vi "Equivalent Circuit.vi"(0 "VISA resource name":refnum<visa-resource-name>, 1 "Equivalent Circuit (0:A)":u32(ring) items=["A", "B", "C", "D", "E"], 2 "Equivalent Circuit Page (T:Not Displaying)":bool=TRUE, 5 "R (1.0 ohm)":dbl=1.0 min=-1e-36 max=9.99999e+37 format="%^.3e", 7 "L (1,0E-6 H)":dbl=1e-06 min=-1e-36 max=1e+38 format="%^.3e", 9 "Ca (1,0E-6 F)":dbl=1e-06 min=-1e-36 max=1e+38 format="%^.3e", 11 "error in (no error)":errorcluster, 12 "Cb (1,0E-6 F)":dbl=1e-06 max=1e+38 format="%^.3e") -> (4 "VISA resource name out":refnum<visa-resource-name>, 15 "error out":errorcluster)   [LabVIEW 2017, in "Agilent 4194.lvlib"]
doc: "This function sets the equivalent circuit and parameters for this equivalent circuit."
uses:
  Agilent 4194.lvlib
panel:
  # "Not Displaying"
  # "Displaying"
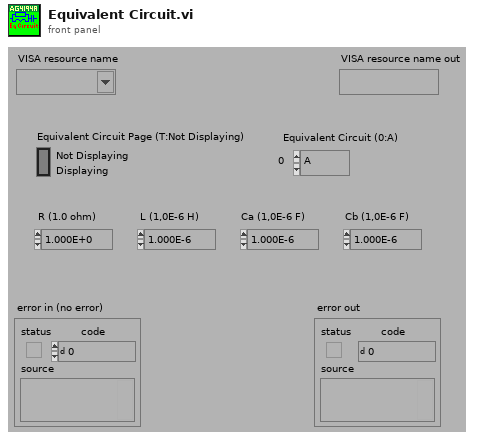
[diagram p1: front panel]
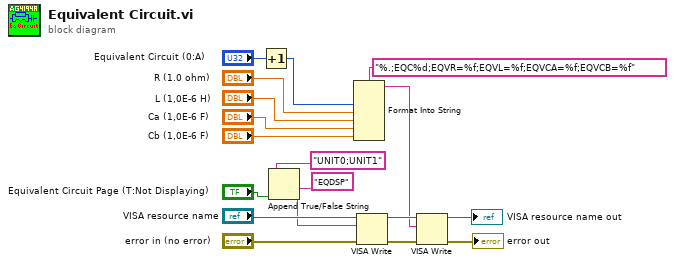
[diagram p0: block diagram]
diagram:
  n1 = Increment(x="Equivalent Circuit (0:A)") -> (x+1=w3:u32)
  n2 = Append True/False String(1:"Equivalent Circuit Page (T:Not Displaying)", 2:"EQDSP", 3:"UNIT0;UNIT1") -> (0:w9:string)  [unwired: 1 in]
  n3 = Format Into String(format string="%.;EQC%d;EQVR=%f;EQVL=%f;EQVCA=%f;EQVCB=%f", w3, "R (1.0 ohm)", "L (1,0E-6 H)", "Ca (1,0E-6 F)", "Cb (1,0E-6 F)") -> (resulting string=w4:string)  [unwired: 2 in, 1 out]
  n4 = VISA Write(VISA resource name="VISA resource name", write buffer=w9, error in (no error)="error in (no error)") -> (VISA resource name out=w8:refnum<visa-resource-name>, error out=w7:errorcluster)  [unwired: 1 out]
  n5 = VISA Write(VISA resource name=w8, write buffer=w4, error in (no error)=w7) -> (VISA resource name out=→"VISA resource name out":refnum<visa-resource-name>, error out=→"error out":errorcluster)  [unwired: 1 out]
